vi "Agilent 34401 Read Single Measurement for all.vi"() -> ()   [LabVIEW 2021]
doc: "This example shows how to configure a measurement and take a single reading."
uses:
  <vilib>/Utility/error.llb/DialogType.ctl
  <instrlib>/Agilent 34401/Public/Configure/Configure Temperature (RTD).vi
  <instrlib>/Agilent 34401/Public/Data/Read (Single Point).vi
  <vilib>/express/express shared/transition.llb/Dynamic To Waveform Array.vi
  <vilib>/express/express arith-compare/Formula/Block/exnFormulaBlock how many pts in the wave.vi
  <vilib>/express/express shared/ex_Modify Signal Name.vi
  <vilib>/express/express shared/transition.llb/Waveform Array To Dynamic.vi
  <vilib>/express/express arith-compare/Formula/XNode/ExpressFormulaBlockNode.xnode
  <instrlib>/Agilent 34401/Agilent 34401.lvlib
panel:
  out "Ratio":string[][](table)
  in  "Function (0: DC Voltage) 3":u16(ring) items=["DC Voltage", "AC Voltage", "2 - Wire Resistance", "4 - Wire Resistance", "DC Current", "AC Current", "Frequency", "Period", "Continuity", "Diode Checking", "VDC:VDC Ratio", "Temperature", "Capacitance"]
  in  "Manual Range (1.00) 3":dbl=1.0 format="%_3f"
  in  "Manual Resolution (5.5 Digits) 3":dbl(ring)=5.5 items=["4.5"=4.5, "5.5"=5.5, "6.5"=6.5]
  in  "Enable Auto Range (T: Enable) 3":bool=TRUE
  in  "Serial Configuration 3":T1={"Baud Rate"=9600, "Parity"=2, "Data Bits"=7} {"Data Bits" items=["7"=7, "8"=8]; "Parity" items=["None", "Odd", "Even"]; "Baud Rate" items=["300"=300, "600"=600, "1200"=1200, "2400"=2400, "4800"=4800, "9600"=9600, "19200"=19200]}
  in  "VISA resource name 4":refnum<visa-resource-name>
  out "Input voltage":string[][](table)
  out "Measurement 4":dbl
  out "temperture":string[][](table)
  out "output voltage":string[][](table)
  out "Input current":string[][](table)
  in  "Unit (0: Celsius)":u16(ring) items=["C", "F", "K"]
  in  "Wire Mode (1: 4-Wire)":i16(ring)=1 items=["2-Wire", "4-Wire"]
  in  "Enable Offset Compensation (F: Disable)":bool
  in  "VISA resource name 2":refnum<visa-resource-name>
  out "Measurement 2":dbl
  in  "Nominal Resistance (100 ohms)":dbl=100.0
  in  "stop":bool
  in  "Function (0: DC Voltage) 2":u16(ring) items=["DC Voltage", "AC Voltage", "2 - Wire Resistance", "4 - Wire Resistance", "DC Current", "AC Current", "Frequency", "Period", "Continuity", "Diode Checking", "VDC:VDC Ratio", "Temperature", "Capacitance"]
  in  "Manual Range (1.00) 2":dbl=1.0 format="%_3f"
  in  "Manual Resolution (5.5 Digits) 2":dbl(ring)=5.5 items=["4.5"=4.5, "5.5"=5.5, "6.5"=6.5]
  in  "Enable Auto Range (T: Enable) 2":bool=TRUE
  in  "Serial Configuration 2":T1={"Baud Rate"=9600, "Parity"=2, "Data Bits"=7} {"Data Bits" items=["7"=7, "8"=8]; "Parity" items=["None", "Odd", "Even"]; "Baud Rate" items=["300"=300, "600"=600, "1200"=1200, "2400"=2400, "4800"=4800, "9600"=9600, "19200"=19200]}
  out "Measurement 3":dbl
  in  "VISA resource name 3":refnum<visa-resource-name>
  in  "Function (0: DC Voltage)":u16(ring) items=["DC Voltage", "AC Voltage", "2 - Wire Resistance", "4 - Wire Resistance", "DC Current", "AC Current", "Frequency", "Period", "Continuity", "Diode Checking", "VDC:VDC Ratio", "Temperature", "Capacitance"]
  in  "Manual Range (1.00)":dbl=1.0 format="%_3f"
  in  "Manual Resolution (5.5 Digits)":dbl(ring)=5.5 items=["4.5"=4.5, "5.5"=5.5, "6.5"=6.5]
  in  "Enable Auto Range (T: Enable)":bool=TRUE
  in  "Serial Configuration":T1={"Baud Rate"=9600, "Parity"=2, "Data Bits"=7} {"Data Bits" items=["7"=7, "8"=8]; "Parity" items=["None", "Odd", "Even"]; "Baud Rate" items=["300"=300, "600"=600, "1200"=1200, "2400"=2400, "4800"=4800, "9600"=9600, "19200"=19200]}
  out "Measurement":dbl
  in  "VISA resource name":refnum<visa-resource-name>
  # "(c) 2005-2015 National Instruments.  ALL RIGHTS RESERVED."
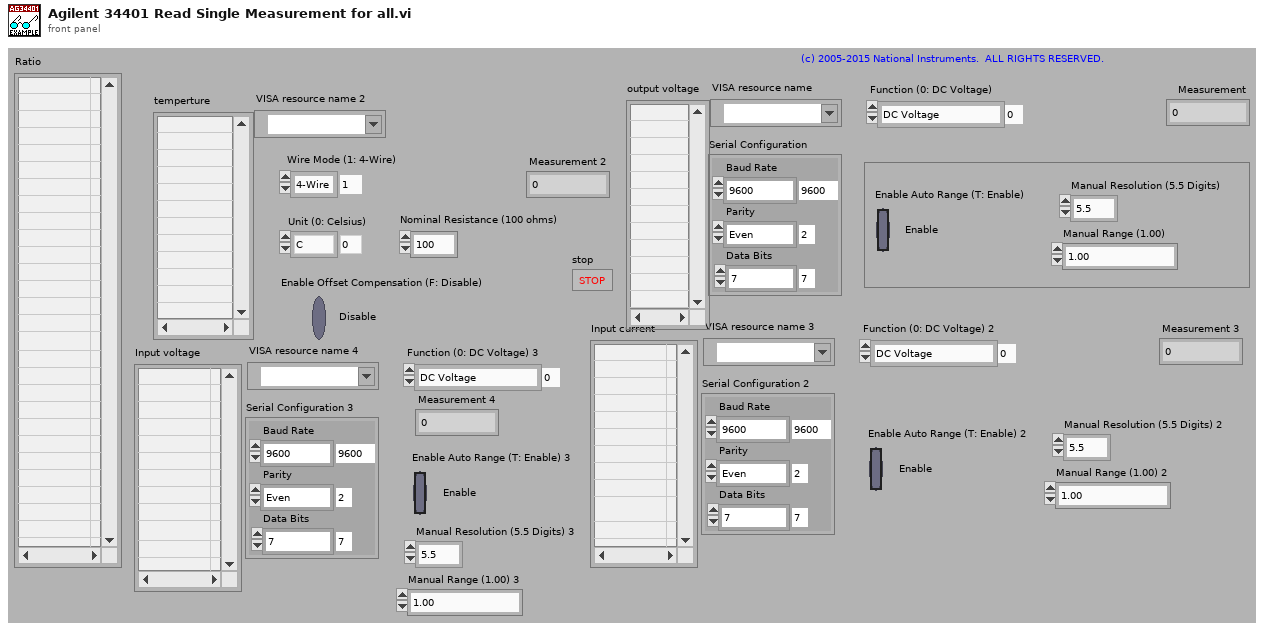
[diagram p1: front panel]
types:
  T1 = cluster{"Baud Rate":u32, "Parity":u16, "Data Bits":u16}
  T2 = typedef "DialogType.ctl" = u16
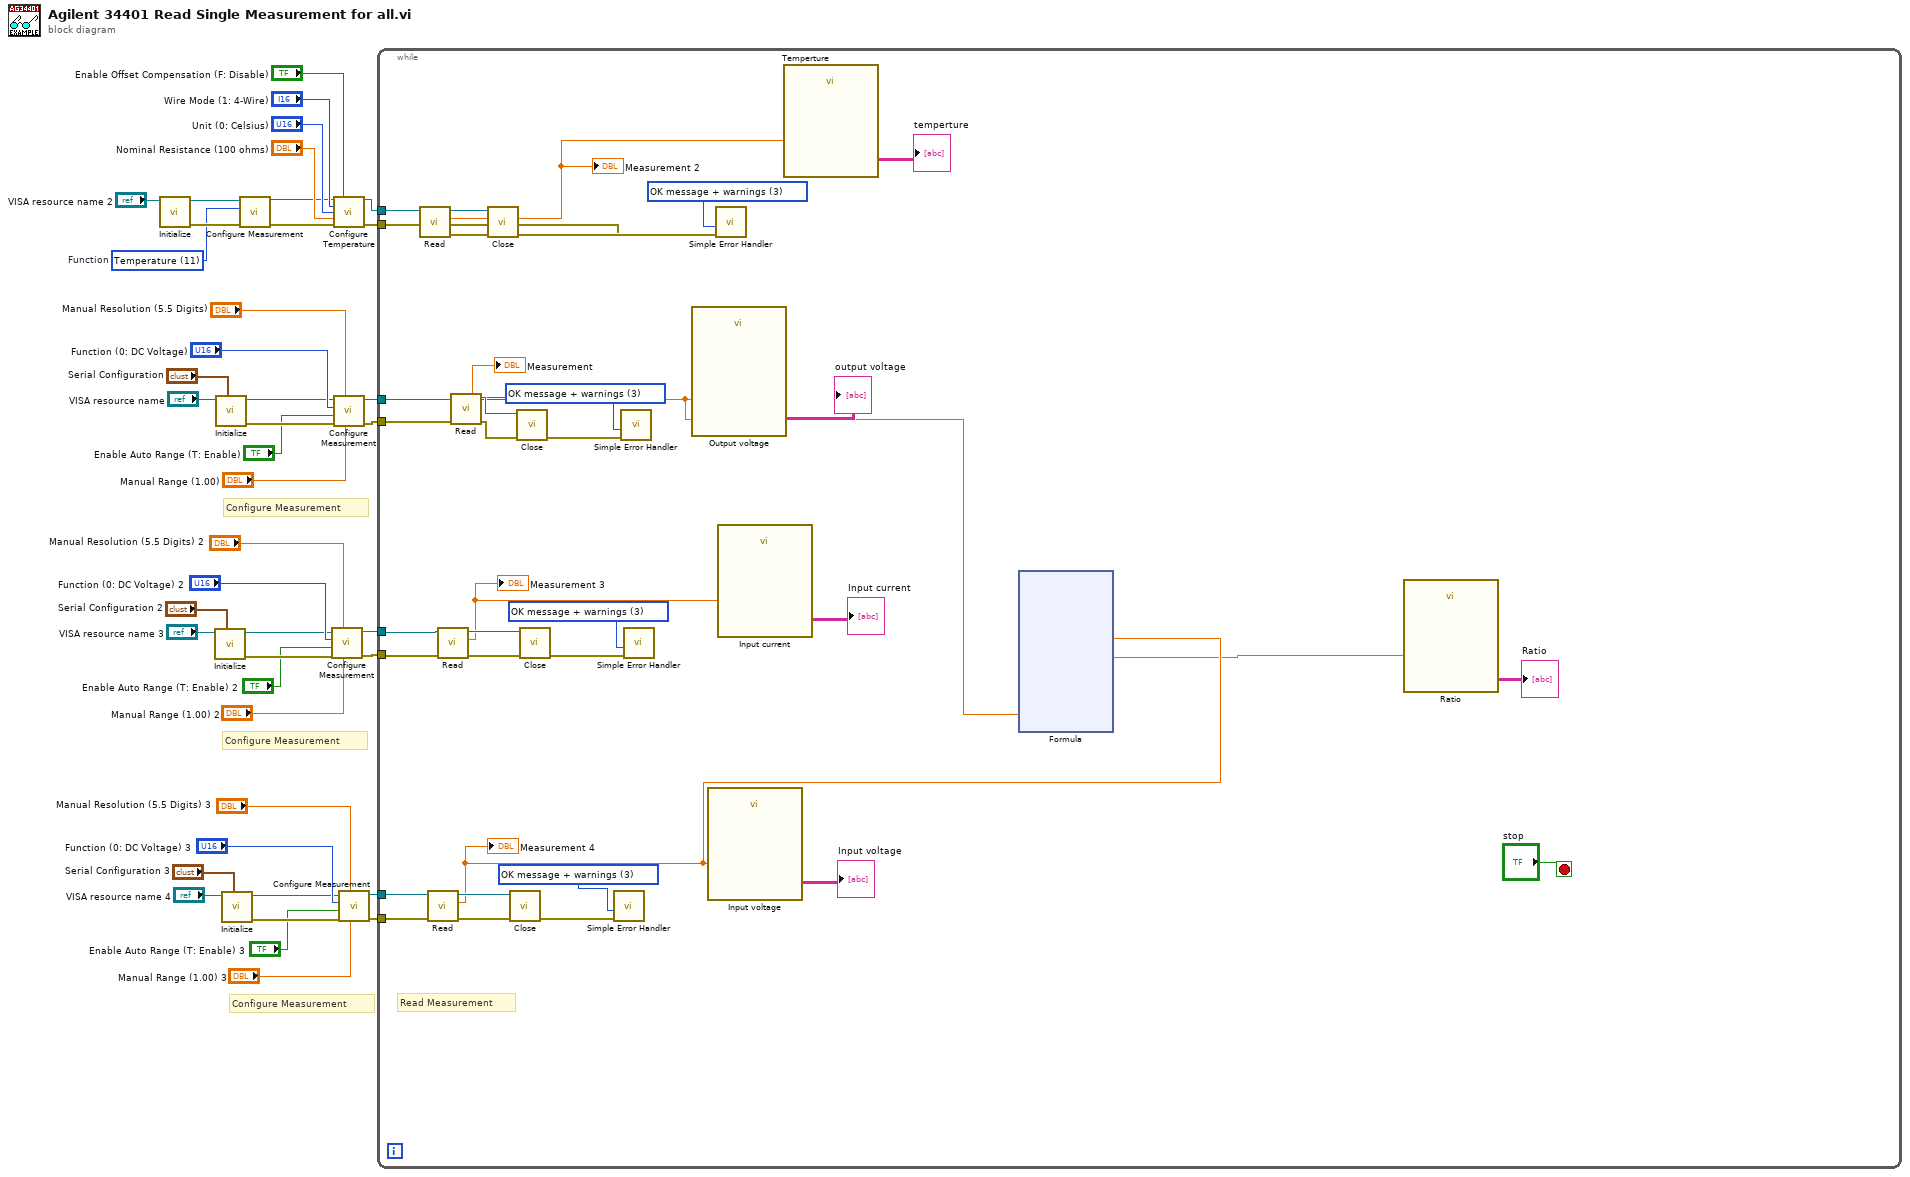
[diagram p0: block diagram]
diagram:
  w13 = u16 11 items=["DC Voltage", "AC Voltage", "2 - Wire Resistance", "4 - Wire Resistance", "DC Current", "AC Current", "Frequency", "Period", "Continuity", "Diode Checking", "VDC:VDC Ratio", "Temperature", "Capacitance"]  # Function
  # "Configure Measurement"
  # "Configure Measurement"
  # "Configure Measurement"
  n1 = call <instrlib>:"Initialize.vi"("VISA resource name"="VISA resource name 2") -> ("error out"=w14:errorcluster, "VISA resource name out"=w15:refnum<visa-resource-name>)  [unwired: 9 in]
  n2 = call <instrlib>:"Initialize.vi"("Serial Configuration"="Serial Configuration 2", "VISA resource name"="VISA resource name 3") -> ("error out"=w28:errorcluster, "VISA resource name out"=w25:refnum<visa-resource-name>)  [unwired: 8 in]
  n3 = call <instrlib>:"Initialize.vi"("Serial Configuration"="Serial Configuration", "VISA resource name"="VISA resource name") -> ("error out"=w36:errorcluster, "VISA resource name out"=w33:refnum<visa-resource-name>)  [unwired: 8 in]
  n4 = call <instrlib>:"Initialize.vi"("Serial Configuration"="Serial Configuration 3", "VISA resource name"="VISA resource name 4") -> ("error out"=w6:errorcluster, "VISA resource name out"=w3:refnum<visa-resource-name>)  [unwired: 8 in]
  n5 = call <instrlib>:"Configure Measurement.vi"("error in (no error)"=w14, "Function (0: DC Voltage)"=w13, "VISA resource name"=w15) -> ("error out"=w16:errorcluster, "VISA resource name out"=w17:refnum<visa-resource-name>)  [unwired: 7 in]
  n6 = call <instrlib>:"Configure Measurement.vi"("Manual Range (1.00)"="Manual Range (1.00) 2", "Manual Resolution (5.5 Digits)"="Manual Resolution (5.5 Digits) 2", "error in (no error)"=w28, "Enable Auto Range (T: Enable)"="Enable Auto Range (T: Enable) 2", "Function (0: DC Voltage)"="Function (0: DC Voltage) 2", "VISA resource name"=w25) -> ("error out"=w24:errorcluster, "VISA resource name out"=w23:refnum<visa-resource-name>)  [unwired: 4 in]
  n7 = call-poly <instrlib>:"Configure Temperature.vi"("VISA resource name"=w17, "Enable Offset Compensation (F: Disable)"="Enable Offset Compensation (F: Disable)", "Wire Mode (1: 4-Wire)"="Wire Mode (1: 4-Wire)", "Unit (0: Celsius)"="Unit (0: Celsius)", "Nominal Resistance (100 ohms)"="Nominal Resistance (100 ohms)", "error in (no error)"=w16) -> ("VISA resource name out"=w12:refnum<visa-resource-name>, "error out"=w11:errorcluster)  [unwired: 8 in]
  n8 = call <instrlib>:"Configure Measurement.vi"("Manual Range (1.00)"="Manual Range (1.00)", "Manual Resolution (5.5 Digits)"="Manual Resolution (5.5 Digits)", "error in (no error)"=w36, "Enable Auto Range (T: Enable)"="Enable Auto Range (T: Enable)", "Function (0: DC Voltage)"="Function (0: DC Voltage)", "VISA resource name"=w33) -> ("error out"=w32:errorcluster, "VISA resource name out"=w31:refnum<visa-resource-name>)  [unwired: 4 in]
  n9 = call <instrlib>:"Configure Measurement.vi"("Manual Range (1.00)"="Manual Range (1.00) 3", "Manual Resolution (5.5 Digits)"="Manual Resolution (5.5 Digits) 3", "error in (no error)"=w6, "Enable Auto Range (T: Enable)"="Enable Auto Range (T: Enable) 3", "Function (0: DC Voltage)"="Function (0: DC Voltage) 3", "VISA resource name"=w3) -> ("error out"=w1:errorcluster, "VISA resource name out"=w2:refnum<visa-resource-name>)  [unwired: 4 in]
  n10 = while {
    tunnel: w32 -> [w68]
    tunnel: w31 -> [w67]
    tunnel: w24 -> [w66]
    tunnel: w23 -> [w65]
    tunnel: w12 -> [w60]
    tunnel: w11 -> [w59]
    tunnel: w2 -> [w49]
    tunnel: w1 -> [w48]
    stop <- "stop" stop-if-true
    w50 = T2 3 items=["no dialog", "OK message", "continue or stop message", "OK message + warnings", "continue/stop + warnings"] ("type of dialog (OK msg:1)")
    w61 = T2 3 items=["no dialog", "OK message", "continue or stop message", "OK message + warnings", "continue/stop + warnings"] ("type of dialog (OK msg:1)")
    w70 = T2 3 items=["no dialog", "OK message", "continue or stop message", "OK message + warnings", "continue/stop + warnings"] ("type of dialog (OK msg:1)")
    w74 = T2 3 items=["no dialog", "OK message", "continue or stop message", "OK message + warnings", "continue/stop + warnings"] ("type of dialog (OK msg:1)")
    # "Read Measurement"
    n11 = call-poly <instrlib>:"Read.vi"("error in (no error)"=w59, "VISA resource name"=w60) -> ("error out"=w64:errorcluster, "Measurement"=w58:dbl, "VISA resource name out"=w63:refnum<visa-resource-name>)  [unwired: 7 in]
    "Measurement 2" <- w58
    n12 = call-poly <instrlib>:"Read.vi"("error in (no error)"=w48, "VISA resource name"=w49) -> ("error out"=w52:errorcluster, "Measurement"=w45:dbl, "VISA resource name out"=w53:refnum<visa-resource-name>)  [unwired: 7 in]
    "Measurement 4" <- w45
    n13 = call-poly <instrlib>:"Read.vi"("error in (no error)"=w66, "VISA resource name"=w65) -> ("error out"=w72:errorcluster, "Measurement"=w46:dbl, "VISA resource name out"=w71:refnum<visa-resource-name>)  [unwired: 7 in]
    "Measurement 3" <- w46
    n14 = call-poly <instrlib>:"Read.vi"("error in (no error)"=w68, "VISA resource name"=w67) -> ("error out"=w76:errorcluster, "Measurement"=w47:dbl, "VISA resource name out"=w75:refnum<visa-resource-name>)  [unwired: 7 in]
    "Measurement" <- w47
    n15 = call <instrlib>:"Close.vi"("error in (no error)"=w64, "VISA resource name"=w63) -> ("error out"=w62:errorcluster)  [unwired: 9 in]
    n16 = call <instrlib>:"Close.vi"("error in (no error)"=w52, "VISA resource name"=w53) -> ("error out"=w51:errorcluster)  [unwired: 9 in]
    n17 = call <instrlib>:"Close.vi"("error in (no error)"=w76, "VISA resource name"=w75) -> ("error out"=w77:errorcluster)  [unwired: 9 in]
    n18 = call <instrlib>:"Close.vi"("error in (no error)"=w72, "VISA resource name"=w71) -> ("error out"=w73:errorcluster)  [unwired: 9 in]
    n19 = call <vilib>:"Simple Error Handler.vi"("type of dialog (OK msg:1)"=w50, "error in (no error)"=w51) -> ()  [unwired: 3 in, 5 out]
    n20 = call <vilib>:"Simple Error Handler.vi"("type of dialog (OK msg:1)"=w74, "error in (no error)"=w77) -> ()  [unwired: 3 in, 5 out]
    n21 = call <vilib>:"Simple Error Handler.vi"("type of dialog (OK msg:1)"=w70, "error in (no error)"=w73) -> ()  [unwired: 3 in, 5 out]
    n22 = call "Output voltage"("Signals"=w47) -> ("Table"=→"output voltage":string[][])  [unwired: 4 in, 6 out]
    n23 = call "Input voltage"("Signals"=w45) -> ("Table"=→"Input voltage":string[][])  [unwired: 4 in, 6 out]
    n24 = call <vilib>:"Simple Error Handler.vi"("type of dialog (OK msg:1)"=w61, "error in (no error)"=w62) -> ()  [unwired: 3 in, 5 out]
    n25 = call "Input current"("Signals"=w46) -> ("Table"=→"Input current":string[][])  [unwired: 4 in, 6 out]
    n26 = call "Temperture"("Signals"=w58) -> ("Table"=→"temperture":string[][])  [unwired: 4 in, 6 out]
    n27 = xnode "Formula"("Input voltage"=w45, "Output voltage"=w47) -> ("结果"=w44:dbl)  [unwired: 1 in, 1 out]
    n28 = call "Ratio"("Signals"=w44) -> ("Table"=→"Ratio":string[][])  [unwired: 4 in, 6 out]
  }
